vi "RSZVB Recall Limit Line.vi"(8 "error in (no error)":errorcluster {"code" format="%.0x"}, 9 "File Name (Trc1.limit)":string="Trc1.limit", 10 "Trace Name (Trc1)":string="Trc1", 11 "VISA session":refnum<visa-resource-name>) -> (0 "error out":errorcluster {"code" format="%.0x"}, 3 "dup VISA session":refnum<visa-resource-name>)   [LabVIEW 2011]
doc: "This VI loads a limit line definition from a specified file and assigns it to a trace with a specified name. Limit lines are created using the CALCulte<Ch/Tr>:LIMit... commands.\n\nRemote-control command(s):\nMMEMory:LOAD:LIMit '<trc_name>','<file_name>'"
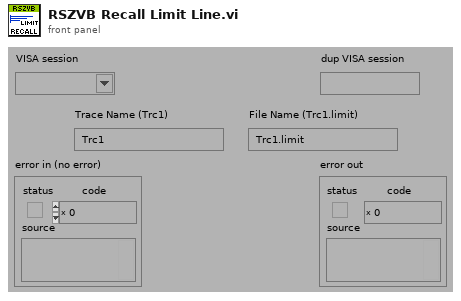
[diagram p1: front panel]
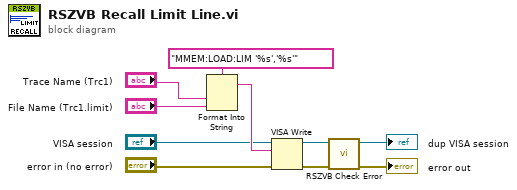
[diagram p0: block diagram]
diagram:
  n1 = Format Into String(format string="MMEM:LOAD:LIM '%s','%s'", "Trace Name (Trc1)", "File Name (Trc1.limit)") -> (resulting string=w7:string)  [unwired: 2 in, 1 out]
  n2 = VISA Write(VISA resource name="VISA session", write buffer=w7, error in (no error)="error in (no error)") -> (VISA resource name out=w9:refnum<visa-resource-name>, error out=w10:errorcluster)  [unwired: 1 out]
  n3 = call "RSZVB Check Error.vi"("error in (no error)"=w10, "VISA session"=w9) -> ("error out"=→"error out":errorcluster, "dup VISA session"=→"dup VISA session":refnum<visa-resource-name>)  [unwired: 8 in]
